vi "실습 9-2.vi"() -> ()   [LabVIEW 2014]
uses:
  <vilib>/Analysis/NI_AALBase.lvlib
panel:
  in  "파일 경로(대화 상자 사용)":path
  out "웨이브폼 그래프":dbl[][](graph)
  out "텍스트":string
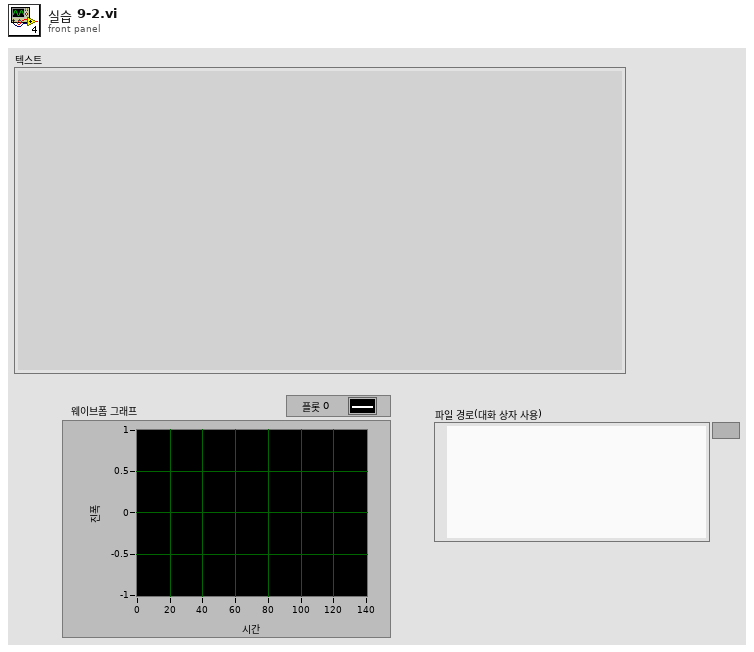
[diagram p1: front panel]
types:
  T1 = enum16{"open", "replace", "create", "open or create", "replace or create", "replace or create with confirmation"}
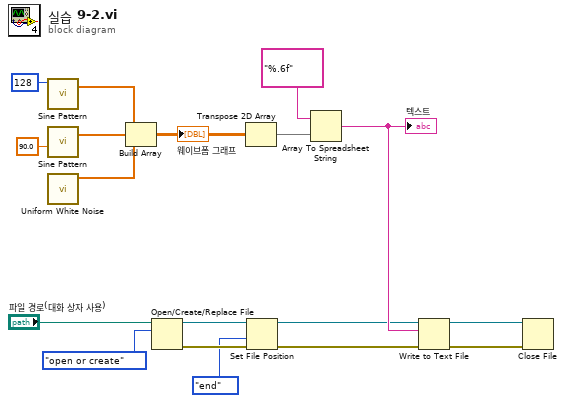
[diagram p0: block diagram]
diagram:
  n1 = call <vilib>:"Sine Pattern.vi"("samples"=128) -> ("Sinusoidal Pattern"=w13:dbl[])  [unwired: 3 in, 1 out]
  n2 = call <vilib>:"Sine Pattern.vi"("phase(degrees)"=90.0) -> ("Sinusoidal Pattern"=w12:dbl[])  [unwired: 3 in, 1 out]
  n3 = call <vilib>:"Uniform White Noise.vi"() -> ("uniform white noise"=w11:dbl[])  [unwired: 10 in, 1 out]
  n4 = Build Array(w13, w12, w11) -> (w10:dbl[][])
  "웨이브폼 그래프" <- w10
  n5 = Open/Create/Replace File(file path (use dialog)="파일 경로(대화 상자 사용)", operation (0:open)=T1."open or create" ("동작(0:open)")) -> (refnum out=w5:refnum<file>, error out=w3:errorcluster)  [unwired: 4 in, 1 out]
  n6 = Transpose 2D Array(2D array=w10) -> (transposed array=w7:dbl[][])
  n7 = Set File Position(refnum=w5, from (0:start)=enum16{"start", "end", "current"}."end" ("시작(0:시작)"), error in=w3) -> (refnum out=w4:refnum<file>, error out=w2:errorcluster)  [unwired: 1 in]
  n8 = Array To Spreadsheet String(array=w7, 3:"%.6f" ("포맷 문자열")) -> (spreadsheet string=w9:string)  [unwired: 1 in]
  "텍스트" <- w9
  n9 = Write to Text File(file (use dialog)=w4, text=w9, error in=w2) -> (refnum out=w17:refnum<file>, error out=w16:errorcluster)  [unwired: 1 in, 1 out]
  n10 = Close File(refnum=w17, error in=w16) -> ()  [unwired: 2 out]
